vi "uView_fp.open.vi"(8 "error in (no error)":errorcluster, 11 "uView Transport":refnum<class "uTransport_uActor.lvclass">) -> (0 "error out":errorcluster)   [LabVIEW 2021, in "uFramework_pack_uActor.lvlib" / "uView.lvclass"]
doc: "Open the FP in a standalone Window."
uses:
  Bin/uFramework.lvlibp/uTransport_uActor/uTransport_uActor.lvclass
  uView.lvclass
  uView.lvclass/uView.ctl
  Bin/uFramework.lvlibp/uActor/uActor.lvclass
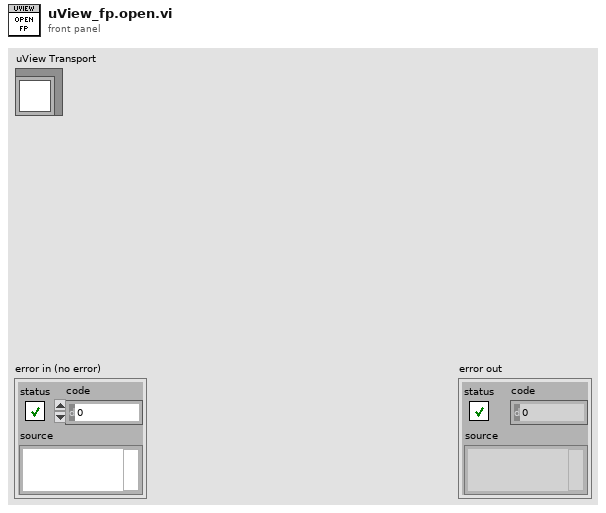
[diagram p1: front panel]
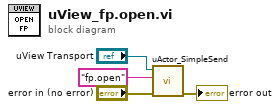
[diagram p0: block diagram]
diagram:
  n1 = call "uActor_SimpleSend.vi"("error in (no error)"="error in (no error)", "Msg"="fp.open", "uActor Transport"="uView Transport") -> ("error out"=→"error out":errorcluster)  [unwired: 8 in]
